vi "Run Measure Logic and Get Results.vi"(8 "error in":errorcluster, 9 "measure call context in":refnum<class "Measure Call Context.lvclass">, 10 "measurement configuration":variant, 11 "measurement logic vi path":path) -> (0 "error out":errorcluster, 1 "measurement error":errorcluster, 2 "measure call context out":refnum<class "Measure Call Context.lvclass">, 3 "measurement output":variant)   [LabVIEW 2020, in "Measurement Plugin Measurement Server.lvlib" / "IMeasurement Service.lvclass"]
uses:
  IMeasurement Service.lvclass
  Measure Call Context/Measure Call Context.lvclass
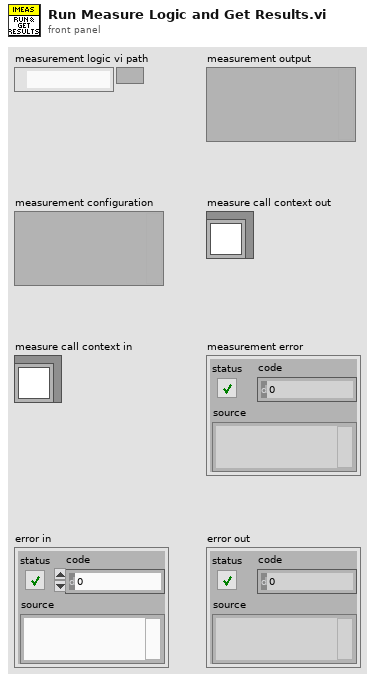
[diagram p1: front panel]
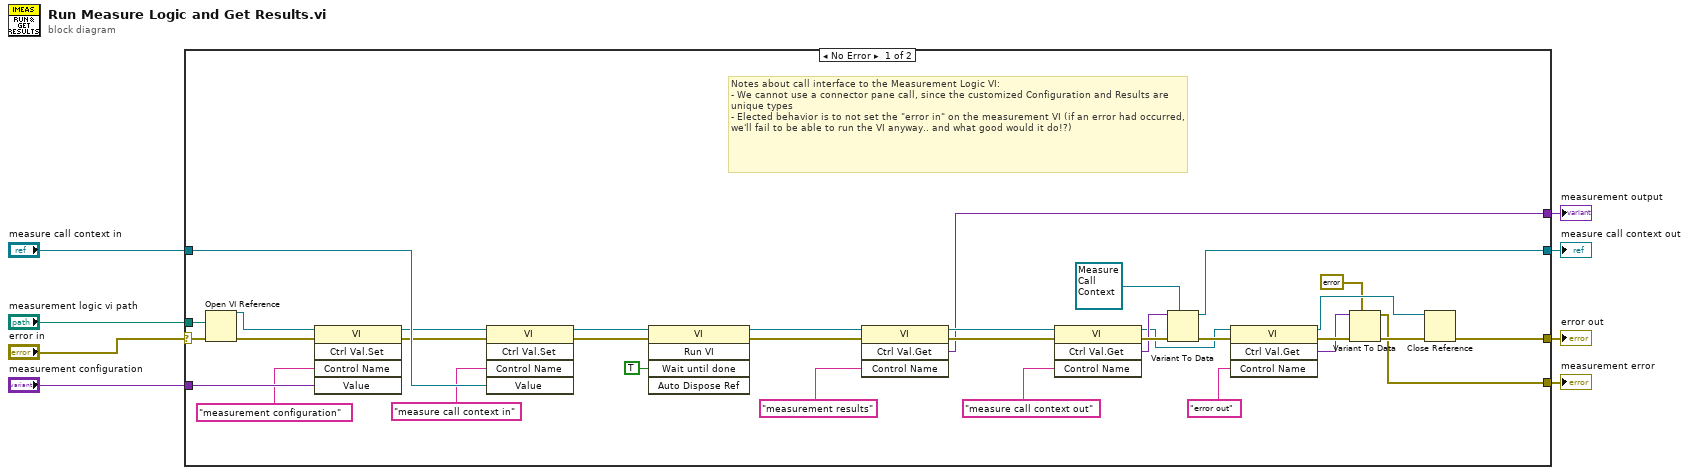
[diagram p0: block diagram]
diagram:
  n1 = case shown="No Error" "error in" {
    selector: "error in" -> [w31 w43]
    tunnel: [w42 w44] -> w8
    tunnel: "measure call context in" -> [w34 w44]
    tunnel: "measurement logic vi path" -> [w33 _]
    tunnel: [w32 _] -> w5
    tunnel: "measurement configuration" -> [w30 _]
    tunnel: [w9 w43] -> w2
    tunnel: [w10 _] -> w1
    frame No Error {
      # "Notes about call interface to the Measurement Logic VI:\n- We cannot use a connector pane call, since the customized Configuration and Results are unique types\n- Elected behavior is to not set the \"error in\" on the measurement VI (if an error had occurred, we'll fail to be able to run the VI anyway.. and what good would it do!?)"
      n2 = Open VI Reference(vi path=w33, error in (no error)=w31) -> (vi reference=w14:refnum<vi>, error out=w15:errorcluster)  [unwired: 4 in]
      n3 = invoke class="VI" method="Ctrl Val.Set"(reference=w14, error in=w15, "Control Name"="measurement configuration", "Value"=w30) -> (reference out=w17:refnum<vi>, error out=w18:errorcluster)  [unwired: 1 in, 3 out]
      n4 = invoke class="VI" method="Ctrl Val.Set"(reference=w17, error in=w18, "Control Name"="measure call context in", "Value"=w34) -> (reference out=w21:refnum<vi>, error out=w20:errorcluster)  [unwired: 1 in, 3 out]
      n5 = invoke class="VI" method="Run VI"(reference=w21, error in=w20, "Wait until done"=TRUE ("Wait Until Done")) -> (reference out=w23:refnum<vi>, error out=w24:errorcluster)  [unwired: 2 in, 3 out]
      n6 = invoke class="VI" method="Ctrl Val.Get"(reference=w23, error in=w24, "Control Name"="measurement results") -> (reference out=w35:refnum<vi>, error out=w37:errorcluster, "Get Control Value Variant"=w32:variant)  [unwired: 1 in, 1 out]
      n7 = invoke class="VI" method="Ctrl Val.Get"(reference=w35, error in=w37, "Control Name"="measure call context out") -> (reference out=w36:refnum<vi>, error out=w40:errorcluster, "Get Control Value Variant"=w39:variant)  [unwired: 1 in, 1 out]
      n8 = Variant To Data(error in=w40, type=refnum<class "Measure Call Context.lvclass"> refnum ("MeasurementContext in"), Variant=w39) -> (data=w42:refnum<class "Measure Call Context.lvclass">, error out=w41:errorcluster)
      n9 = invoke class="VI" method="Ctrl Val.Get"(reference=w36, error in=w41, "Control Name"="error out") -> (reference out=w27:refnum<vi>, error out=w28:errorcluster, "Get Control Value Variant"=w26:variant)  [unwired: 1 in, 1 out]
      n10 = Variant To Data(error in=w28, type=errorcluster {"status"=FALSE, "code"=0, "source"=""} ("error out"), Variant=w26) -> (data=w10:errorcluster, error out=w29:errorcluster)
      n11 = Close Reference(reference=w27, error in (no error)=w29) -> (error out=w9:errorcluster)
    }
    frame Error {
    }
  }
  "measure call context out" <- w8
  "error out" <- w2
  "measurement output" <- w5
  "measurement error" <- w1
